vi "LHF.DB.Mongo.Util.VariantToFields.vi"(0 "projection type":variant, 5 "error in (no error)":errorcluster) -> (14 "BsonDocument":refnum<k24>, 19 "error out":errorcluster)   [LabVIEW 2013, in "LHF.DB.Mongo.lvclass"]
uses:
  LHF.DB.Mongo.lvclass
  C:/Users/Ricardo/Desktop/Projetos/LabVIEW-MongoDB/src/Driver/MongoDB.Bson.dll
  LabVIEW-MongoDB/src/Driver/MongoDB.Bson.dll
  C:/Users/Ricardo/Desktop/Projetos/LabVIEW-MongoDB/src/Driver/MongoDB.Driver.dll
  LabVIEW-MongoDB/src/Driver/MongoDB.Driver.dll
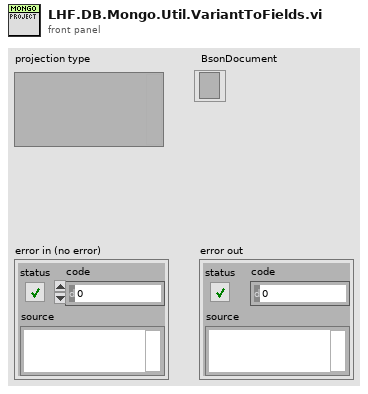
[diagram p1: front panel]
types:
  T1 = typedef "LHF.DB.Mongo.lvclass/LHF.DB.Mongo.Typedef.VariantData.ctl" = cluster{"Type Enum":T2, "Name":string, "Variant":variant}
  T2 = typedef "VariantType.lvlib/Type.ctl" = enum8{"Invalid Type", "Void", "I8", "I16", "I32", "I64", "U8", "U16", "U32", "U64", "Single Float", "Double Float", "Extended Float", "Single Complex", "Double Complex", "Extended Complex", "Enum U8", "Enum U16", "Enum U32", "Enum U64", "Single Float With Unit", "Double Float With Unit", "Extended Float With Unit", "Single Complex with Unit", "Double Complex with Unit", "Extended Complex with Unit", "Boolean", "String", "Path", "Picture", "Tag", "Array", "Cluster", "Variant", "LV Variant", "Waveform", "Timestamp", "Digital Waveform", "Digital Data", "ExpressData", "Refnum", "External Data", "VI", "Poly VI", "LabVIEW Class Instance", "Fixed Point"}
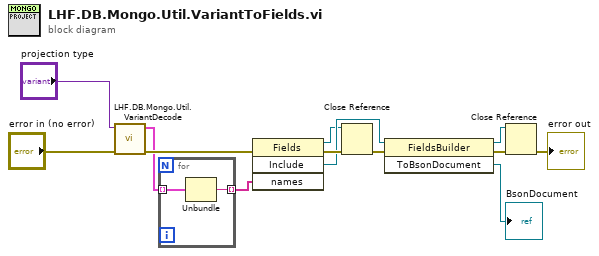
[diagram p0: block diagram]
diagram:
  n1 = call "LHF.DB.Mongo.Util.VariantDecode.vi"("error in (no error)"="error in (no error)", "variant"="projection type") -> ("error out"=w13:errorcluster, "Variant Data"=w9:T1[])  [unwired: 7 in, 1 out]
  n2 = for {
    tunnel: w9 -> [w15] mode=indexing
    tunnel: [w14] -> w10 mode=indexing
    n3 = Unbundle(w15) -> ("Name"=w14:string)  [unwired: 2 out]
  }
  n4 = invoke class="Fields" method="Include"(error in=w13, "names"=w10) -> (reference out=w4:refnum<k24>, error out=w7:errorcluster, "Include"=w6:refnum<k24>)  [unwired: 2 in, 1 out]
  n5 = Close Reference(reference=w4, error in (no error)=w7) -> (error out=w5:errorcluster)
  n6 = invoke class="FieldsBuilder" method="ToBsonDocument"(reference=w6, error in=w5) -> (reference out=w3:refnum<k24>, error out=w8:errorcluster, "ToBsonDocument"=→"BsonDocument":refnum<k24>)  [unwired: 1 in]
  n7 = Close Reference(reference=w3, error in (no error)=w8) -> (error out=→"error out":errorcluster)
